vi "Save Collimation Steps Data.vi"(4 "Data":dbl[][](array[numeric]), 6 "Item":string[](array[string]), 8 "Error In":errorcluster, 10 "SN":string, 11 "路径":string="C:\\BeamViewImage\\Collimation Steps Data") -> (0 "error out":errorcluster caption="错误输出")   [LabVIEW 2018]
uses:
  <vilib>/Utility/file.llb/Write Delimited Spreadsheet (string).vi
  <vilib>/Utility/file.llb/Write Delimited Spreadsheet (DBL).vi
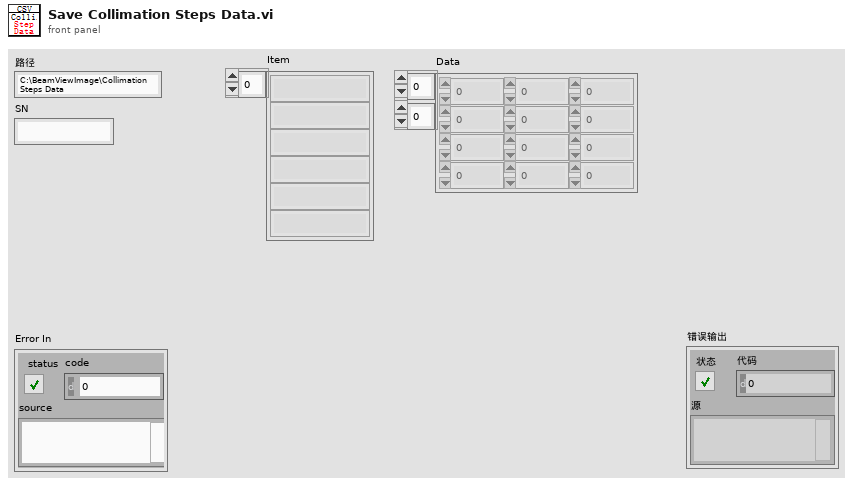
[diagram p1: front panel]
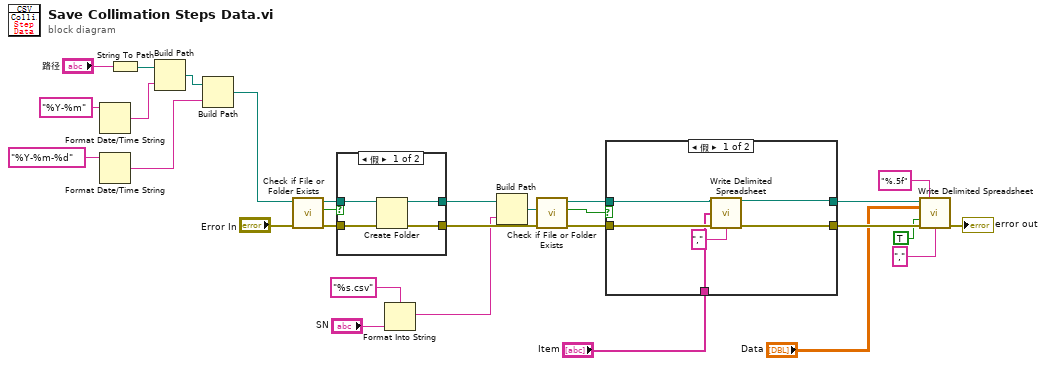
[diagram p0: block diagram]
diagram:
  n1 = Format Date/Time String(time format string (%c)="%Y-%m") -> (date/time string=w15:string)  [unwired: 2 in]
  n2 = Format Date/Time String(time format string (%c)="%Y-%m-%d") -> (date/time string=w13:string)  [unwired: 2 in]
  n3 = String To Path(string="路径") -> (path=w16:path)
  n4 = Build Path(base path=w16, name or relative path=w15) -> (appended path=w29:path)
  n5 = Build Path(base path=w29, name or relative path=w13) -> (appended path=w2:path)
  n6 = call <vilib>:"Check if File or Folder Exists.vi"("error in (no error)"="Error In", "path"=w2) -> ("error out"=w26:errorcluster, "file or folder exists?"=w27:bool, "dup path"=w24:path)  [unwired: 7 in]
  n7 = case shown="假" w27 {
    tunnel: w26 -> [w32 w34]
    tunnel: w24 -> [w33 w35]
    tunnel: [w31 w35] -> w21
    tunnel: [w30 w34] -> w23
    frame False {
      n8 = Create Folder(path (use dialog)=w33, error in=w32) -> (created path=w31:path, error out=w30:errorcluster)  [unwired: 1 in, 1 out]
    }
    frame True {
    }
  }
  n9 = Format Into String(format string="%s.csv" ("格式字符串"), "SN") -> (resulting string=w10:string)  [unwired: 2 in, 1 out]
  n10 = Build Path(base path=w21, name or relative path=w10) -> (appended path=w22:path)
  n11 = call <vilib>:"Check if File or Folder Exists.vi"("error in (no error)"=w23, "path"=w22) -> ("error out"=w18:errorcluster, "file or folder exists?"=w20:bool, "dup path"=w19:path)  [unwired: 7 in]
  n12 = case shown="假" w20 {
    tunnel: w19 -> [w41 w43]
    tunnel: w18 -> [w39 w42]
    tunnel: [w40 w43] -> w9
    tunnel: [w38 w42] -> w8
    tunnel: "Item" -> [w37 _]
    frame False {
      n13 = call-poly <vilib>:"Write Delimited Spreadsheet.vi"("file path (dialog if empty)"=w41, "1D data"=w37, "error in (no error)"=w39, "delimiter (\\t)"="," ("delimiter (\\t)")) -> ("new file path (Not A Path if cancelled)"=w40:path, "error out"=w38:errorcluster)  [unwired: 10 in]
    }
    frame True {
    }
  }
  n14 = call-poly <vilib>:"Write Delimited Spreadsheet.vi"("file path (dialog if empty)"=w9, "format (%.3f)"="%.5f" ("format (%s)"), "2D data"="Data", "append to file? (new file:F)"=TRUE, "error in (no error)"=w8, "delimiter (\\t)"="," ("delimiter (\\t)")) -> ("error out"=→"error out":errorcluster)  [unwired: 8 in, 1 out]
